vi "Read Result.vi"(8 "error in (no error)":errorcluster, 11 "ControlDragEndedMsg In":refnum<class "ControlDragEndedMsg.lvclass">) -> (0 "error out":errorcluster, 2 "Result":enum16{"Drop Cancel", "Drop Move", "Drop Copy"}(ring), 3 "ControlDragEndedMsg Out":refnum<class "ControlDragEndedMsg.lvclass">)   [LabVIEW 2018, in "MVA Framework.lvlib" / "ActorEvents.lvlib" / "ControlDragEndedMsg.lvclass"]
uses:
  ControlDragEndedMsg.lvclass
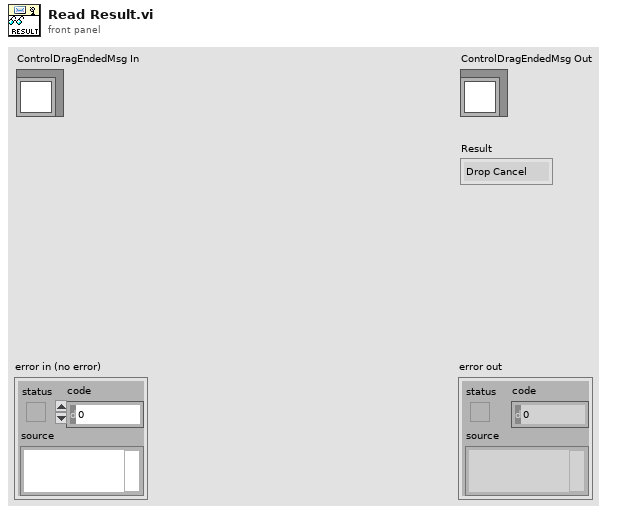
[diagram p1: front panel]
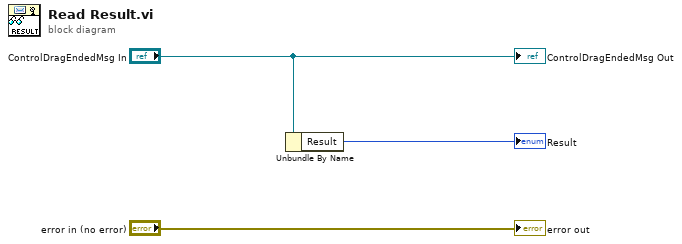
[diagram p0: block diagram]
diagram:
  n1 = Unbundle By Name("ControlDragEndedMsg In") -> ("Result"=→"Result":enum16{"Drop Cancel", "Drop Move", "Drop Copy"})
  "error out" <- "error in (no error)"
  "ControlDragEndedMsg Out" <- "ControlDragEndedMsg In"
